vi "DataTreeCtrl moveFile.vi"(8 "error in (no error)":errorcluster, 11 "DataTreeCtrl in":refnum<class "DataTreeCtrl.lvclass">) -> (0 "error out":errorcluster, 3 "DataTreeCtrl out":refnum<class "DataTreeCtrl.lvclass">)   [LabVIEW 2018, in "DataTreeCtrl.lvclass"]
uses:
  DataTreeCtrl.lvclass
  DataTreeCtrl.lvclass/DataTreeCtrl.ctl
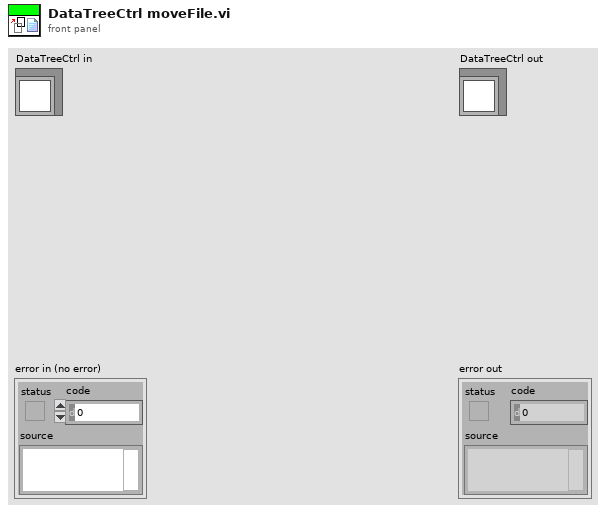
[diagram p1: front panel]
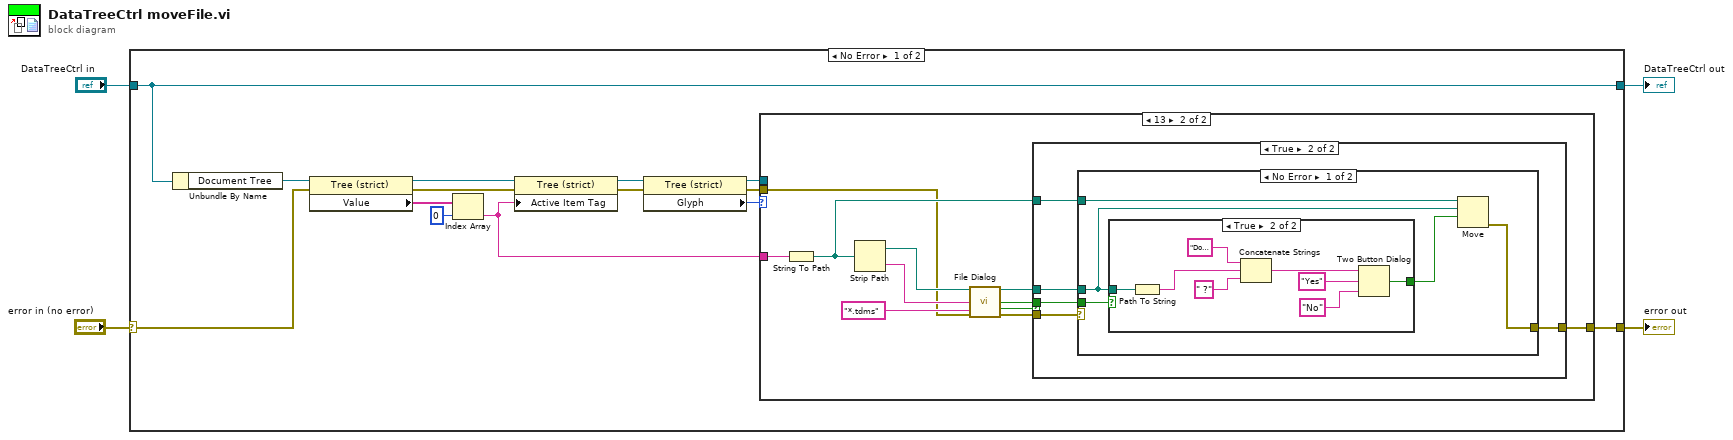
[diagram p0: block diagram]
diagram:
  n1 = case shown="No Error" "error in (no error)" {
    selector: "error in (no error)" -> [w6 w52]
    tunnel: [w5 w52] -> w3
    tunnel: [w18 w51] -> w1
    tunnel: "DataTreeCtrl in" -> [w18 w51]
    frame No Error {
      n2 = Unbundle By Name(w18) -> ("Document Tree"=w11:refnum<vi>)
      n3 = property class="Tree (strict)"(reference=w11, error in=w6) -> (reference out=w17:refnum<vi>, error out=w14:errorcluster, "Value"=w16:string[])
      n4 = Index Array(array=w16, index=0) -> (element=w7:string)
      n5 = property class="Tree (strict)"(reference=w17, error in=w14, "Active Item Tag"=w7) -> (reference out=w13:refnum<vi>, error out=w12:errorcluster)
      n6 = property class="Tree (strict)"(reference=w13, error in=w12) -> (reference out=w9:refnum<vi>, error out=w8:errorcluster, "Glyph"=w10:i32)
      n7 = case shown="13" w10 {
        tunnel: w9 -> [_ _]
        tunnel: w8 -> [w19 w20]
        tunnel: w7 -> [_ w30]
        tunnel: [w19 w21] -> w5
        frame 14, Default {
        }
        frame 13 {
          n8 = String To Path(string=w30) -> (path=w25:path)
          n9 = Strip Path(path=w25) -> (stripped path=w29:path, name=w28:string)
          n10 = call "File Dialog"("start path"=w29, "default name"=w28, "error in"=w20, "pattern (all files)"="*.tdms") -> ("selected path"=w24:path, "exists"=w26:bool, "cancelled"=w23:bool, "error out"=w22:errorcluster)  [unwired: 8 in]
          n11 = case shown="True" w23 {
            tunnel: w26 -> [_ w36]
            tunnel: w25 -> [_ w35]
            tunnel: w24 -> [_ w34]
            tunnel: w22 -> [w31 w33]
            tunnel: [w31 w32] -> w21
            frame False {
            }
            frame True {
              n12 = case shown="No Error" w33 {
                selector: w33 -> [_ w50]
                tunnel: w36 -> [w41 _]
                tunnel: w35 -> [w40 _]
                tunnel: w34 -> [w39 _]
                tunnel: [w38 w50] -> w32
                frame No Error {
                  n13 = case shown="True" w41 {
                    tunnel: w39 -> [_ w49]
                    tunnel: [_ w42] -> w37
                    frame False {
                    }
                    frame True {
                      n14 = Path To String(path=w49) -> (string=w46:string)
                      n15 = Concatenate Strings("Do you want overwrite " ("message"), w46, " ?" ("string")) -> (w45:string)
                      n16 = Two Button Dialog(message=w45, 1:"No" ("F button name (\"Cancel\")"), 2:"Yes" ("T button name (\"OK\")")) -> (T button?=w42:bool)
                    }
                  }
                  n17 = Move(source path=w40, 9:w37, 10:w39) -> (error out=w38:errorcluster)  [unwired: 2 in, 2 out]
                }
                frame Error {
                }
              }
            }
          }
        }
      }
    }
    frame Error {
    }
  }
  "error out" <- w3
  "DataTreeCtrl out" <- w1
